vi "Initialize Database Change UI Tree.vi"(8 "error in (no error)":errorcluster, 10 "VS Filtered Change List":T1 {"Incoming"."Missing"."Node Ref" format="%.0x"; "Incoming"."Changed"."Old"."Node Ref" format="%.0x"; "Outgoing"."Missing"."Node Ref" format="%.0x"; "Outgoing"."Changed"."Old"."Node Ref" format="%.0x"}, 11 "TreeControl in":refnum<vi>) -> (0 "error out":errorcluster, 3 "TreeControl out":refnum<vi>)   [LabVIEW 2025, in "Protection and Counter Addon System Explorer.lvlib"]
uses:
  Protection and Counter Addon System Explorer.lvlib
  Types/Filtered XNET Changes.ctl
  Types/Database Changes.ctl
  Types/Base Frame Info_NoVS.ctl
  Types/Signal Attributes.ctl
  Types/CAN Filter Type.ctl
  Types/Base Frame Info.ctl
  <vilib>/NI VeriStand/Custom Device API/Custom Device Item Ref.ctl
  Types/Related CAN Frames.ctl
  Types/Related CAN Frames No VS.ctl
  <vilib>/NI VeriStand/Custom Device API/Custom Device API.lvlib
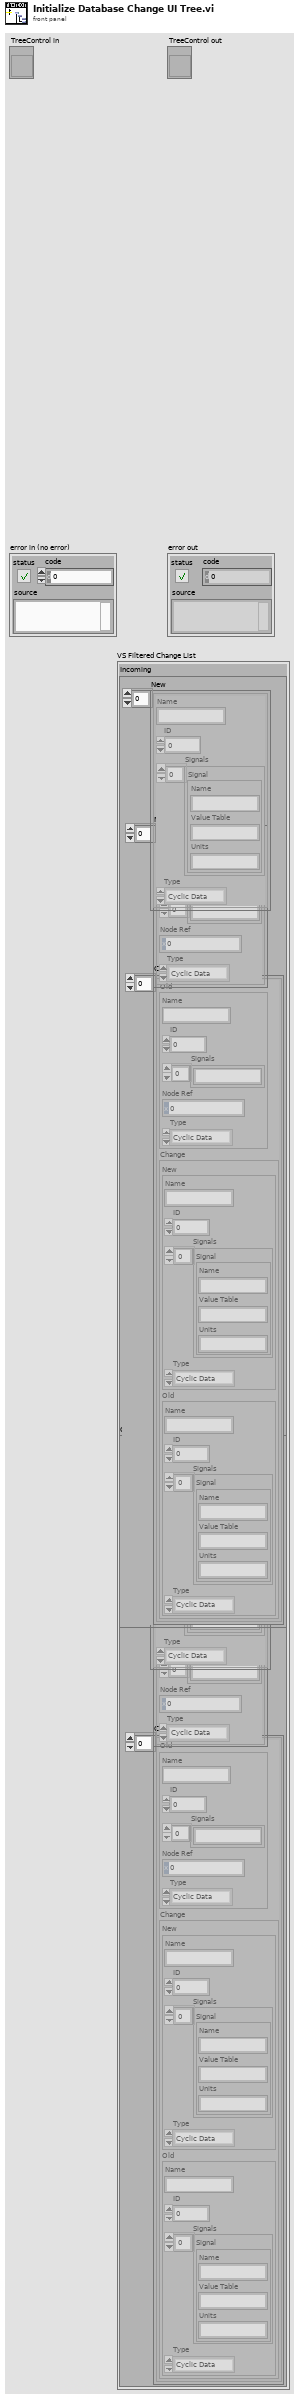
[diagram p1: front panel]
types:
  T1 = typedef "Protection and Counter Addon System Explorer.lvlib/Filtered XNET Changes.ctl" = cluster{"Incoming":T2, "Outgoing":T2}
  T2 = typedef "Protection and Counter Addon System Explorer.lvlib/Database Changes.ctl" = cluster{"New":T3[], "Missing":T6[], "Changed":T8[]}
  T3 = typedef "Protection and Counter Addon System Explorer.lvlib/Base Frame Info_NoVS.ctl" = cluster{"Name":string, "ID":u32, "Signals":T4[], "Type":T5}
  T4 = typedef "Protection and Counter Addon System Explorer.lvlib/Signal Attributes.ctl" = cluster{"Name":string, "Value Table":string, "Units":string}
  T5 = typedef "Protection and Counter Addon System Explorer.lvlib/CAN Filter Type.ctl" = enum16{"Cyclic Data", "Event Data", "Cyclic/Event", "All"}
  T6 = typedef "Protection and Counter Addon System Explorer.lvlib/Base Frame Info.ctl" = cluster{"Name":string, "ID":u32, "Signals":string[], "Node Ref":T7, "Type":T5}
  T7 = typedef "Custom Device API.lvlib/Custom Device Item Ref.ctl" = u64
  T8 = typedef "Protection and Counter Addon System Explorer.lvlib/Related CAN Frames.ctl" = cluster{"Old":T6, "Change":T9}
  T9 = typedef "Protection and Counter Addon System Explorer.lvlib/Related CAN Frames No VS.ctl" = cluster{"New":T3, "Old":T3}
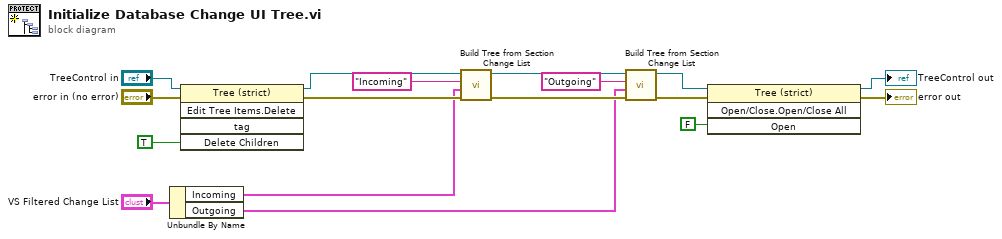
[diagram p0: block diagram]
diagram:
  n1 = Unbundle By Name("VS Filtered Change List") -> ("Incoming"=w8:T2, "Outgoing"=w3:T2)
  n2 = invoke on="Invoke Node" class="Tree (strict)" method="Edit Tree Items.Delete"(reference="TreeControl in", error in="error in (no error)", "Delete Children"=TRUE ("Delete Children?")) -> (reference out=w11:refnum<vi>, error out=w10:errorcluster)  [unwired: 2 in, 3 out]
  n3 = call "Build Tree from Section Change List.vi"("error in (no error)"=w10, "Database Changes"=w8, "Section"="Incoming", "TreeControl in"=w11) -> ("error out"=w4:errorcluster, "TreeControl out"=w6:refnum<vi>)  [unwired: 6 in]
  n4 = call "Build Tree from Section Change List.vi"("error in (no error)"=w4, "Database Changes"=w3, "Section"="Outgoing", "TreeControl in"=w6) -> ("error out"=w1:errorcluster, "TreeControl out"=w5:refnum<vi>)  [unwired: 6 in]
  n5 = invoke on="Invoke Node" class="Tree (strict)" method="Open/Close.Open/Close All"(reference=w5, error in=w1, "Open"=FALSE ("Open?")) -> (reference out=→"TreeControl out":refnum<vi>, error out=→"error out":errorcluster)  [unwired: 1 in, 2 out]
